vi "CI_IMAQ_Close.vi"(11 "Camera data":variant) -> ()   [LabVIEW 2011]
uses:
  GenericIMAQCameraInstance.ctl
  Main/Camera/GenericCameraConfigType.ctl
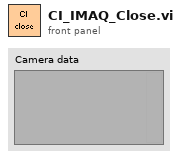
[diagram p1: front panel]
types:
  T1 = typedef "GenericIMAQCameraInstance.ctl" = cluster{"Session":refnum<k11>, "Settings":T2}
  T2 = typedef "GenericCameraConfigType.ctl" = cluster{"Framerate (Hz)":i32, "Exposure time (us)":i32, "Image size":cluster{"Width":i32, "Height":i32}, "Number of buffers":i32}
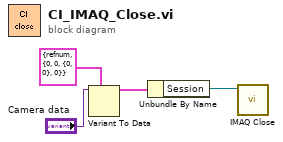
[diagram p0: block diagram]
diagram:
  n1 = Variant To Data(type=T1 {"Session"=refnum, "Settings"={"Framerate (Hz)"=0, "Exposure time (us)"=0, "Image size"={"Width"=0, "Height"=0}, "Number of buffers"=0}} ("Camera data 2"), Variant="Camera data") -> (data=w2:T1)  [unwired: 1 in, 1 out]
  n2 = Unbundle By Name(w2) -> ("Session"=w1:refnum<k11>)
  n3 = call <vilib>:"IMAQ Close.vi"("IMAQ Session In"=w1) -> ()  [unwired: 10 in, 1 out]
